vi "Get Pixel.vi"   [LabVIEW 2011, in "labvvis.lvlib"]
doc: "Returns the value of a pixel in an image."
uses:
  <userlib>/labvvis/labvvis.lvlib
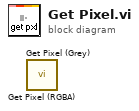
[diagram p0: block diagram]
diagram:
  n1 = call <userlib>:"Get Pixel (RGBA).vi"() -> ()  [unwired: 5 in, 3 out]
  n2 = call <userlib>:"Get Pixel (Grey).vi"() -> ()  [unwired: 5 in, 3 out]
